vi "Recurse Through OPC Items.vi"(6 "LUT":variant, 8 "error in (no error)":errorcluster, 9 "Parent Tag":string, 10 "reference out":refnum<vi>, 11 "OPC UA Client Ref":refnum<k21>) -> (0 "error out":errorcluster, 3 "OPC UA Client Ref":refnum<k21>, 4 "LUT":variant)   [LabVIEW 2013, in "OPC UA Client System Explorer.lvlib"]
uses:
  OPC UA Client System Explorer.lvlib
  <vilib>/OPCUA/NI OPC UA Client.lvlib
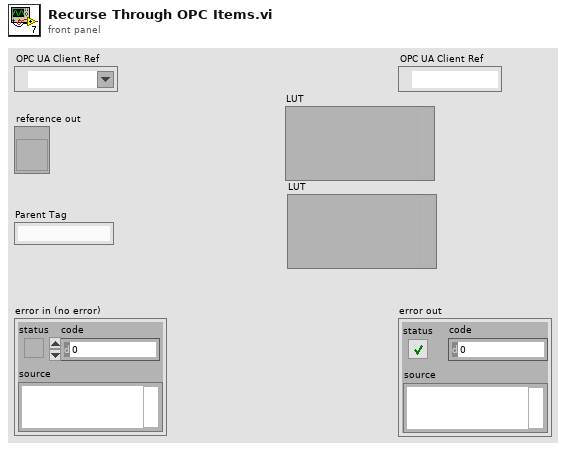
[diagram p1: front panel]
types:
  T1 = cluster{"node path":string, "node name":string, "node type":enum32{"Other", "Folder", "Item/Property"}}[]
  T2 = cluster{"name":string, "node type":enum32{"Other", "Folder", "Item/Property"}, "DataType":u32, "access":enum16{"Null", "Read", "Write", "Read&Write"}, "description":string}
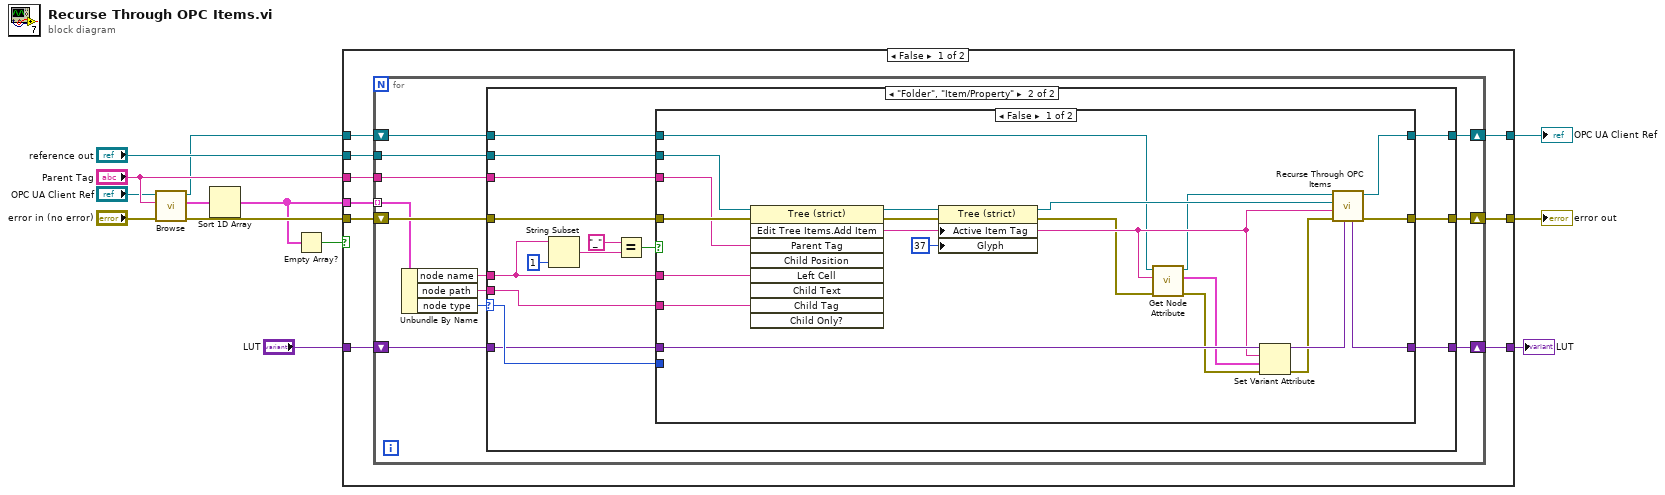
[diagram p0: block diagram]
diagram:
  n1 = call <vilib>:"Browse.vi"("error in (no error)"="error in (no error)", "node path"="Parent Tag", "OPC UA client refnum in"="OPC UA Client Ref") -> ("error out"=w13:errorcluster, "browse result"=w11:T1, "OPC UA client refnum out"=w5:refnum<k21>)  [unwired: 5 in, 1 out]
  n2 = Sort 1D Array(array=w11) -> (sorted array=w1:T1)
  n3 = Empty Array?(array=w1) -> (empty?=w10:bool)
  n4 = case shown="False" w10 {
    tunnel: w13 -> [w22 w79]
    tunnel: "reference out" -> [w21 _]
    tunnel: [w20 w79] -> w7
    tunnel: "Parent Tag" -> [w19 _]
    tunnel: w1 -> [w18 _]
    tunnel: w5 -> [w17 w78]
    tunnel: [w16 w78] -> w4
    tunnel: [w15 w77] -> w3
    tunnel: "LUT" -> [w14 w77]
    frame False {
      n5 = for {
        tunnel: w18 -> [w33] mode=indexing
        tunnel: w19 -> [w29]
        shift-right: [w28] -> w20
        shift-left: w22 -> [w34]
        tunnel: w21 -> [w30]
        shift-right: [w26] -> w16
        shift-left: w17 -> [w27]
        shift-right: [w24] -> w15
        shift-left: w14 -> [w23]
        n6 = Unbundle By Name(w33) -> ("node name"=w32:string, "node path"=w31:string, "node type"=w25:enum32{"Other", "Folder", "Item/Property"})
        n7 = case shown="\"Folder\", \"Item/Property\"" w25 {
          selector: w25 -> [_ w40]
          tunnel: w34 -> [w37 w52]
          tunnel: w32 -> [_ w45]
          tunnel: w31 -> [_ w51]
          tunnel: w30 -> [_ w50]
          tunnel: w29 -> [_ w49]
          tunnel: [w37 w48] -> w28
          tunnel: w27 -> [w36 w47]
          tunnel: [w36 w46] -> w26
          tunnel: [w35 w39] -> w24
          tunnel: w23 -> [w35 w38]
          frame "Other" {
          }
          frame "Folder", "Item/Property" {
            n8 = String Subset(string=w45, length (rest)=1 ("length (rest)")) -> (substring=w43:string)  [unwired: 1 in]
            n9 = Equal?(x="_", y=w43) -> (x = y?=w41:bool)
            n10 = case shown="False" w41 {
              tunnel: w52 -> [w73 w76]
              tunnel: w51 -> [w72 _]
              tunnel: w50 -> [w71 _]
              tunnel: w49 -> [w70 _]
              tunnel: [w69 w76] -> w48
              tunnel: w47 -> [w55 w75]
              tunnel: [w68 w75] -> w46
              tunnel: w45 -> [w67 _]
              tunnel: w40 -> [_ _]
              tunnel: [w60 w74] -> w39
              tunnel: w38 -> [w62 w74]
              frame False {
                n11 = invoke class="Tree (strict)" method="Edit Tree Items.Add Item"(reference=w71, error in=w73, "Parent Tag"=w70, "Left Cell"=w67, "Child Tag"=w72) -> (reference out=w65:refnum<vi>, error out=w66:errorcluster, "Edit Tree Items:Add Item"=w58:string)  [unwired: 4 in, 6 out]
                n12 = property class="Tree (strict)"(reference=w65, error in=w66, "Active Item Tag"=w58, "Glyph"=37 ("Active Item:Symbol Index")) -> (reference out=w64:refnum<vi>, error out=w57:errorcluster)
                n13 = call <vilib>:"Get Node Attribute.vi"("error in (no error)"=w57, "node path"=w58, "OPC UA client refnum in"=w55) -> ("error out"=w56:errorcluster, "node attribute"=w53:T2, "OPC UA client refnum out"=w54:refnum<k21>)  [unwired: 6 in]
                n14 = Set Variant Attribute(Variant=w62, name=w58, value=w53, error in=w56) -> (Variant out=w61:variant, error out=w59:errorcluster)  [unwired: 1 out]
                n15 = call "Recurse Through OPC Items.vi"("LUT"=w61, "error in (no error)"=w59, "Parent Tag"=w58, "reference out"=w64, "OPC UA Client Ref"=w54) -> ("error out"=w69:errorcluster, "OPC UA Client Ref"=w68:refnum<k21>, "LUT"=w60:variant)  [unwired: 4 in]
              }
              frame True {
              }
            }
          }
        }
      }
    }
    frame True {
    }
  }
  "OPC UA Client Ref" <- w4
  "error out" <- w7
  "LUT" <- w3
